vi "home_position_change.vi"(10 "Position":dbl[](array[numeric]), 11 "Dist. b/w cells line":dbl[](array[numeric])) -> (3 "Array":dbl[](array[numeric]))   [LabVIEW 2021]
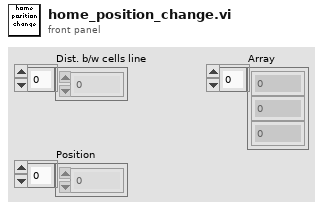
[diagram p1: front panel]
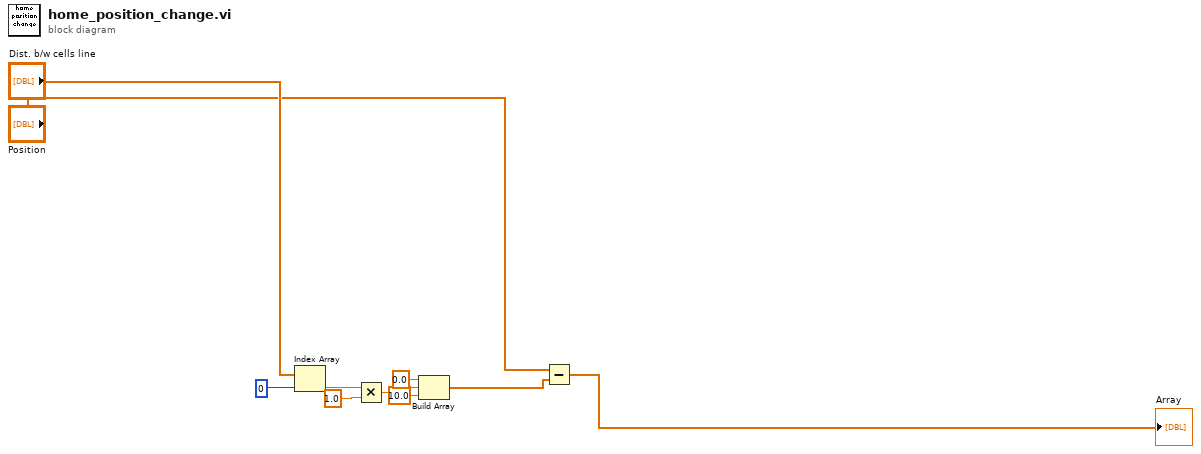
[diagram p0: block diagram]
diagram:
  n1 = Index Array(array="Dist. b/w cells line", index=0) -> (element=w8:dbl)
  n2 = Multiply(x=w8, y=1.0) -> (x*y=w10:dbl)
  n3 = Build Array(0.0 ("element"), w10, 10.0 ("element")) -> (w7:dbl[])
  n4 = Subtract(x="Position", y=w7) -> (x-y=→"Array":dbl[])
